vi "p2.vi"() -> ()   [LabVIEW 2023, in "d21.lvlib"]
uses:
  d21.lvlib
  AOC/AOC.lvlib
panel:
  in  "Steps":u64=26501365
  out "Answer":u64=628206330073385
  in  "Example":string="...........\n.....###.#.\n.###.##..#.\n..#.#...#..\n....#.#....\n.##..S####.\n.##..#...#.\n.......##..\n.##.#.####.\n.##..##.##.\n..........."
  in  "Example":bool
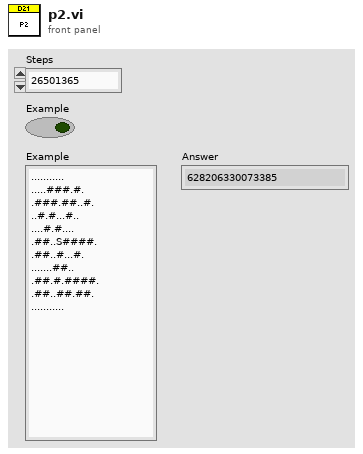
[diagram p1: front panel]
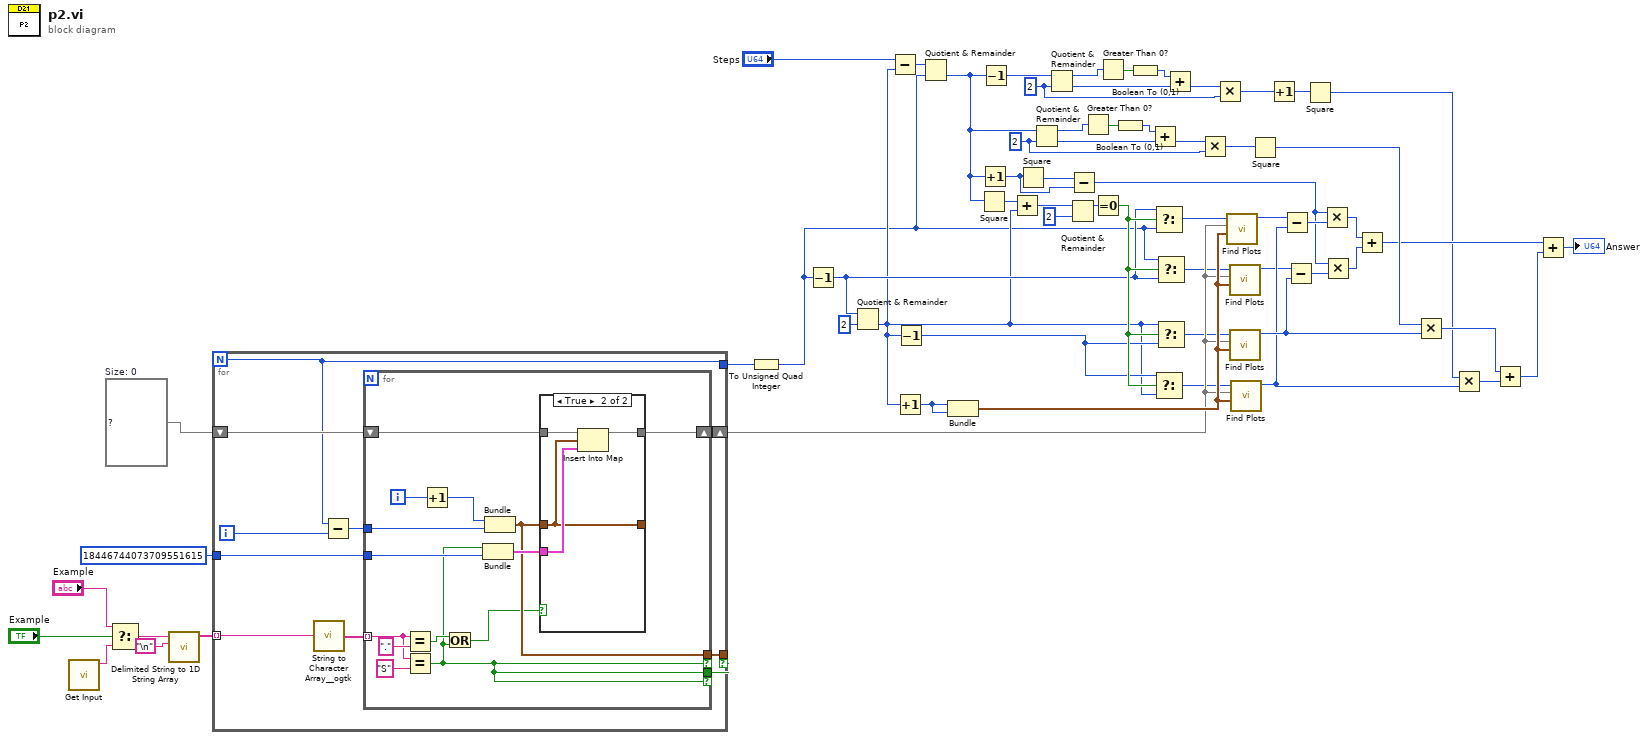
[diagram p0: block diagram]
diagram:
  w47 = u64 2 ("y")
  w50 = u64 2 ("y")
  w25 = map{cluster{i32, i32}, cluster{bool, u64}} {}  # Size: 0
  n1 = call "Get Input.vi"() -> ("Input"=w63:string)  [unwired: 11 in]
  n2 = Select(t="Example", s="Example", f=w63) -> (s? t:f=w58:string)
  n3 = call <vilib>:"Delimited String to 1D String Array.vi"("delimiter"="\n", "delimited string"=w58) -> ("string array"=w24:string[])  [unwired: 9 in]
  n4 = for {
    N -> [w65]
    tunnel: w24 -> [w64] mode=indexing
    tunnel: [w71] -> _ if=w70
    tunnel: u64 18446744073709551615 -> [w69]
    shift-right: [w67] -> w27
    shift-left: w25 -> [w68]
    tunnel: [w65] -> w5
    i -> [w72]
    n5 = call <userlib>:"String to Character Array__ogtk.vi"("Input String"=w64) -> ("Character Array"=w73:string[])
    n6 = Subtract(x=w65, y=w72) -> (x-y=w66:i32)
    n7 = for {
      tunnel: w73 -> [w86] mode=indexing
      tunnel: w66 -> [w83]
      tunnel: [w77] -> w71 if=w75
      tunnel: [w75] -> w70 if=w75
      tunnel: w69 -> [w82]
      shift-right: [w81] -> w67
      shift-left: w68 -> [w80]
      i -> [w84]
      n8 = Equal?(x=w86, y=".") -> (x = y?=w76:bool)
      n9 = Equal?(x=w86, y="S") -> (x = y?=w75:bool)
      n10 = Increment(x=w84) -> (x+1=w78:i32)
      n11 = Or(x=w76, y=w75) -> (x .or. y?=w74:bool)
      n12 = Bundle(w75, w82) -> (w79:cluster{bool, u64})  [unwired: 1 in]
      n13 = Bundle(w78, w83) -> (w77:cluster{i32, i32})  [unwired: 1 in]
      n14 = case shown="True" w74 {
        tunnel: [w89 w93] -> w81
        tunnel: w80 -> [w89 w92]
        tunnel: w77 -> [w88 w90]
        tunnel: w79 -> [_ w91]
        tunnel: [w88 w90] -> _
        frame False {
        }
        frame True {
          n15 = Insert Into Map(map in=w92, key=w90, value=w91) -> (map out=w93:map{cluster{i32, i32}, cluster{bool, u64}})  [unwired: 2 out]
        }
      }
    }
  }
  n16 = To Unsigned Quad Integer(1:w5) -> (0:w1:u64)
  n17 = Decrement(x=w1) -> (x-1=w7:u64)
  n18 = Quotient & Remainder(x=w7, y=u64 2) -> (floor(x/y)=w2:u64)  [unwired: 1 out]
  n19 = Subtract(x="Steps", y=w2) -> (x-y=w8:u64)
  n20 = Increment(x=w2) -> (x+1=w9:u64)
  n21 = Decrement(x=w2) -> (x-1=w6:u64)
  n22 = Quotient & Remainder(x=w8, y=w1) -> (floor(x/y)=w4:u64)  [unwired: 1 out]
  n23 = Bundle(w9, w9) -> (w57:cluster{u64, u64})  [unwired: 1 in]
  n24 = Square(x=w4) -> (x^2=w23:u64)
  n25 = Increment(x=w4) -> (x+1=w3:u64)
  n26 = Decrement(x=w4) -> (x-1=w40:u64)
  n27 = Add(x=w23, y=w2) -> (x+y=w18:u64)
  n28 = Square(x=w3) -> (x^2=w39:u64)
  n29 = Quotient & Remainder(x=w4, y=w50) -> (x-y*floor(x/y)=w54:u64, floor(x/y)=w55:u64)
  n30 = Quotient & Remainder(x=w40, y=w47) -> (x-y*floor(x/y)=w43:u64, floor(x/y)=w42:u64)
  n31 = Quotient & Remainder(x=w18, y=u64 2) -> (x-y*floor(x/y)=w16:u64)  [unwired: 1 out]
  n32 = Subtract(x=w39, y=w3) -> (x-y=w20:u64)
  n33 = Greater Than 0?(x=w54) -> (x > 0?=w53:bool)
  n34 = Equal To 0?(x=w16) -> (x = 0?=w12:bool)
  n35 = Greater Than 0?(x=w43) -> (x > 0?=w44:bool)
  n36 = Boolean To (0,1)(Boolean=w53) -> (0, 1=w51:i16)
  n37 = Boolean To (0,1)(Boolean=w44) -> (0, 1=w46:i16)
  n38 = Add(x=w51, y=w55) -> (x+y=w52:u64)
  n39 = Select(t=w7, s=w12, f=w1) -> (s? t:f=w15:u64)
  n40 = Select(t=w6, s=w12, f=w2) -> (s? t:f=w14:u64)
  n41 = Select(t=w1, s=w12, f=w7) -> (s? t:f=w11:u64)
  n42 = Select(t=w2, s=w12, f=w6) -> (s? t:f=w13:u64)
  n43 = Add(x=w46, y=w42) -> (x+y=w45:u64)
  n44 = Multiply(x=w52, y=w50) -> (x*y=w49:u64)
  n45 = Multiply(x=w45, y=w47) -> (x*y=w48:u64)
  n46 = call "Find Plots.vi"("Start"=w57, "Map"=w27, "Steps"=w15) -> ("Answer"=w56:u64)  [unwired: 8 in]
  n47 = call "Find Plots.vi"("Start"=w57, "Map"=w27, "Steps"=w11) -> ("Answer"=w19:u64)  [unwired: 8 in]
  n48 = call "Find Plots.vi"("Start"=w57, "Map"=w27, "Steps"=w13) -> ("Answer"=w36:u64)  [unwired: 8 in]
  n49 = call "Find Plots.vi"("Start"=w57, "Map"=w27, "Steps"=w14) -> ("Answer"=w34:u64)  [unwired: 8 in]
  n50 = Square(x=w49) -> (x^2=w35:u64)
  n51 = Increment(x=w48) -> (x+1=w41:u64)
  n52 = Subtract(x=w56, y=w34) -> (x-y=w38:u64)
  n53 = Subtract(x=w19, y=w36) -> (x-y=w37:u64)
  n54 = Square(x=w41) -> (x^2=w21:u64)
  n55 = Multiply(x=w20, y=w38) -> (x*y=w33:u64)
  n56 = Multiply(x=w20, y=w37) -> (x*y=w32:u64)
  n57 = Add(x=w33, y=w32) -> (x+y=w30:u64)
  n58 = Multiply(x=w35, y=w36) -> (x*y=w22:u64)
  n59 = Multiply(x=w21, y=w34) -> (x*y=w31:u64)
  n60 = Add(x=w22, y=w31) -> (x+y=w29:u64)
  n61 = Add(x=w30, y=w29) -> (x+y=→"Answer":u64)
